vi "is abstract node.vi"(8 "error in":errorcluster, 11 "module editor node in":refnum<class "module editor node.lvclass">) -> (0 "error out":errorcluster, 2 "abstract":bool, 3 "module editor node out":refnum<class "module editor node.lvclass">)   [LabVIEW 2013, in "PL Framework Configuration Tool.lvlib" / "module editor node.lvclass"]
uses:
  module editor node.lvclass
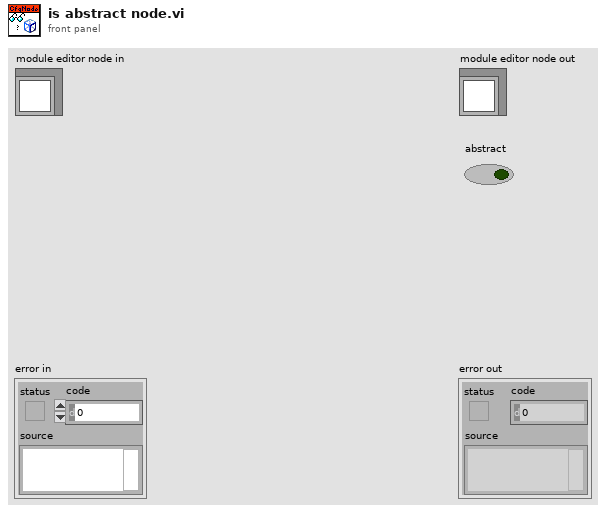
[diagram p1: front panel]
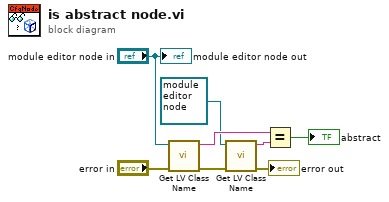
[diagram p0: block diagram]
diagram:
  n1 = call <vilib>:"Get LV Class Name.vi"("error in (no error)"="error in", "object"="module editor node in") -> ("error out"=w6:errorcluster, "class name"=w7:string)  [unwired: 8 in]
  n2 = call <vilib>:"Get LV Class Name.vi"("error in (no error)"=w6, "object"=refnum<class "module editor node.lvclass"> refnum ("module editor node in 2")) -> ("error out"=→"error out":errorcluster, "class name"=w8:string)  [unwired: 8 in]
  n3 = Equal?(x=w7, y=w8) -> (x = y?=→"abstract":bool)
  "module editor node out" <- "module editor node in"
